vi "Save Controls Attribute.vi"(8 "error in (no error)":errorcluster, 10 "Control Refs":refnum<vi>[](array[refnum]), 11 "ScriptsDialogConfiguration in":refnum<class "ScriptsDialogConfiguration.lvclass">) -> (0 "error out":errorcluster, 3 "ScriptsDialogConfiguration out":refnum<class "ScriptsDialogConfiguration.lvclass">)   [LabVIEW 2015, in "ScriptsDialogConfiguration.lvclass"]
uses:
  ScriptsDialogConfiguration.lvclass
  UIConfiguration/UIConfiguration.lvclass/UIConfiguration.ctl
  UIConfiguration/UIConfiguration.lvclass
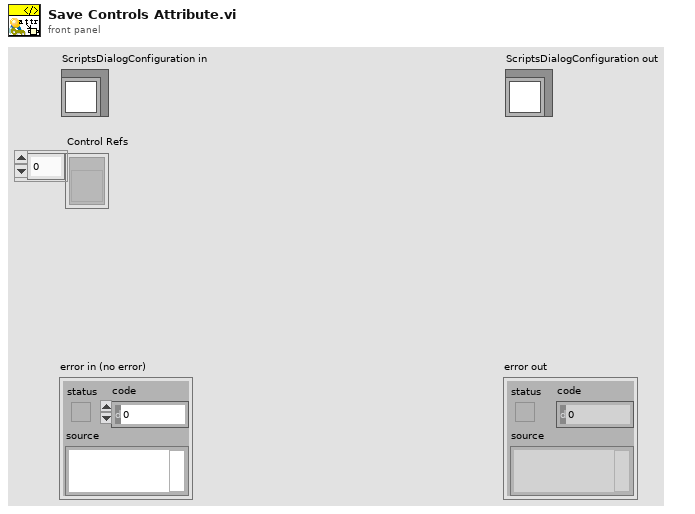
[diagram p1: front panel]
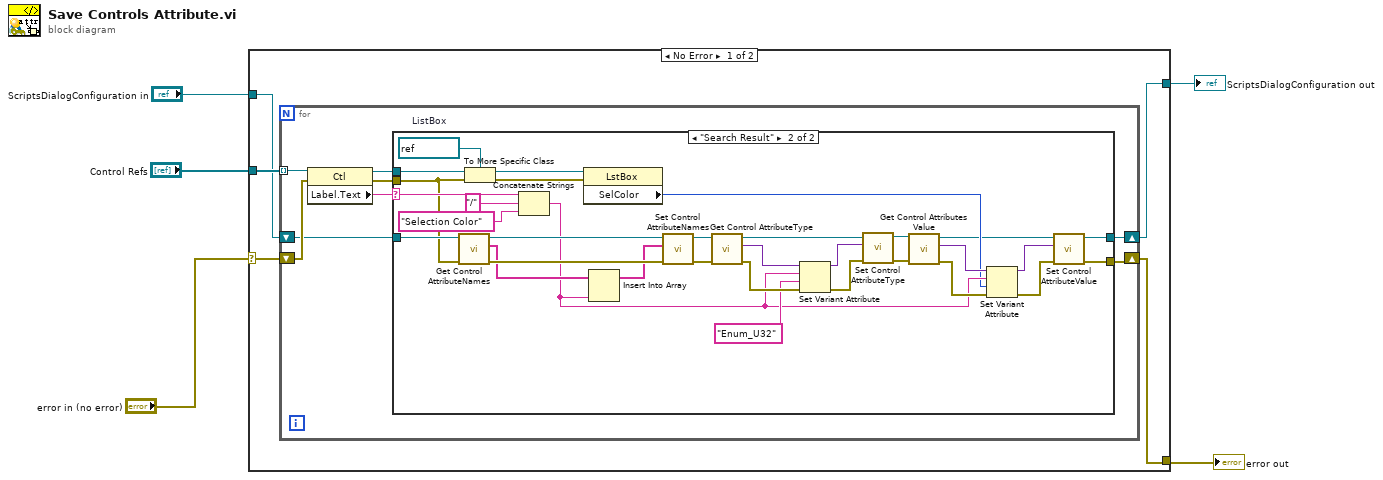
[diagram p0: block diagram]
diagram:
  n1 = case shown="No Error" "error in (no error)" {
    selector: "error in (no error)" -> [w9 w54]
    tunnel: "Control Refs" -> [w10 _]
    tunnel: "ScriptsDialogConfiguration in" -> [w8 w53]
    tunnel: [w7 w53] -> w2
    tunnel: [w6 w54] -> w1
    frame No Error {
      n2 = for {
        tunnel: w10 -> [w18] mode=indexing
        shift-right: [w11] -> w6
        shift-left: w9 -> [w16]
        shift-right: [w12] -> w7
        shift-left: w8 -> [w13]
        n3 = property class="Ctl"(reference=w18, error in=w16) -> (reference out=w14:refnum<vi>, error out=w15:errorcluster, "Label.Text"=w17:string)
        n4 = case shown="\"Search Result\"" w17 {
          selector: w17 -> [_ w51]
          tunnel: w15 -> [w19 w48]
          tunnel: w14 -> [_ w47]
          tunnel: w13 -> [w20 w52]
          tunnel: [w20 w22] -> w12
          tunnel: [w19 w21] -> w11
          frame Default {
          }
          frame "Search Result" {
            w46 = refnum<vi> refnum  # ListBox
            n5 = call "Get Control AttributeNames.vi"("error in (no error)"=w48, "UIConfiguration in"=w52) -> ("error out"=w42:errorcluster, "AttributeNames"=w41:string[], "UIConfiguration out"=w43:refnum<class "ScriptsDialogConfiguration.lvclass">)  [unwired: 7 in]
            n6 = To More Specific Class(target class=w46, reference=w47, error in=w48) -> (specific class reference=w45:refnum<vi>, error out=w44:errorcluster)
            n7 = Concatenate Strings(w51, "/" ("string"), "Selection Color" ("string")) -> (w27:string)
            n8 = property class="LstBox"(reference=w45, error in=w44) -> ("SelColor"=w26:u32)  [unwired: 2 out]
            n9 = Insert Into Array(array=w41, new element=w27) -> (w40:string[])  [unwired: 1 in]
            n10 = call "Set Control AttributeNames.vi"("error in (no error)"=w42, "AttributeNames"=w40, "UIConfiguration in"=w43) -> ("error out"=w38:errorcluster, "UIConfiguration out"=w39:refnum<class "ScriptsDialogConfiguration.lvclass">)  [unwired: 7 in]
            n11 = call "Get Control AttributeType.vi"("error in (no error)"=w38, "UIConfiguration in"=w39) -> ("error out"=w36:errorcluster, "AttributeType"=w37:variant, "UIConfiguration out"=w32:refnum<class "ScriptsDialogConfiguration.lvclass">)  [unwired: 7 in]
            n12 = Set Variant Attribute(Variant=w37, name=w27, value="Enum_U32", error in=w36) -> (Variant out=w33:variant, error out=w34:errorcluster)  [unwired: 1 out]
            n13 = call "Set Control AttributeType.vi"("error in (no error)"=w34, "AttributeType"=w33, "UIConfiguration in"=w32) -> ("error out"=w30:errorcluster, "UIConfiguration out"=w31:refnum<class "ScriptsDialogConfiguration.lvclass">)  [unwired: 7 in]
            n14 = call "Get Control Attributes Value.vi"("error in (no error)"=w30, "UIConfiguration in"=w31) -> ("error out"=w28:errorcluster, "AttributesValue"=w29:variant, "UIConfiguration out"=w23:refnum<class "ScriptsDialogConfiguration.lvclass">)  [unwired: 7 in]
            n15 = Set Variant Attribute(Variant=w29, name=w27, value=w26, error in=w28) -> (Variant out=w25:variant, error out=w24:errorcluster)  [unwired: 1 out]
            n16 = call "Set Control AttributeValue.vi"("error in (no error)"=w24, "AttributeValue"=w25, "UIConfiguration in"=w23) -> ("error out"=w21:errorcluster, "UIConfiguration out"=w22:refnum<class "ScriptsDialogConfiguration.lvclass">)  [unwired: 7 in]
          }
        }
      }
    }
    frame Error {
    }
  }
  "error out" <- w1
  "ScriptsDialogConfiguration out" <- w2
